vi "BioFeedback5(DAQ+FlowControl).vi"(0 "Start Trial":bool, 1 "Moving Average Length (s)":dbl=0.5, 3 "Frames Per Second":dbl=30.0, 4 "Sample rate (Hz)":dbl=1000.0, 5 "End Trial":bool, 9 "Data Directory":path, 11 "End Program":bool, 12 "File Name":string, 13 "VR Data Input File":path=path "C:/Users/Tinggroup/Desktop/VRMuscleActivationVisualizer/StationaryVisualFeedbackVR/assets/BiofeedbackData.txt", 14 "VR Percent Path":path=path "C:/Users/Tinggroup/Desktop/VRMuscleActivationVisualizer/StationaryVisualFeedbackVR/assets/BiofeedbackTargetPercentage.txt") -> (6 "Trial Data":waveform(dbl)(graph), 10 "Moving Avg RMS Graph":dbl(graph), 15 "raw data":dynamicdata(graph))   [LabVIEW 2016]
uses:
  <vilib>/Utility/error.llb/DialogType.ctl
  <vilib>/Analysis/5stat.llb/RMS (DBL).vi
  <vilib>/Waveform/WDTOps.llb/WDT Append Waveforms DBL.vi
  <vilib>/Waveform/WDTFileIO.llb/ Write Waveform to File.vi
  <vilib>/Analysis/NI_AALPro.lvlib
panel:
  in  "Extension":string="_EMG.txt"
  in  "Target Percentage":dbl
  out "Trial Data":waveform(dbl)
  out "Trial In Progress":bool
  in  "Trial Number":dbl
  in  "MARK":bool
  out "Moving Avg RMS":dbl(slide) scale=0.0..2.0
  out "Rectified Moving Average Sample":waveform(dbl)[](graph)
  out "Filtered data":waveform(dbl)
  in  "Lower Cut-Off":dbl=20.0
  in  "Upper Cut-Off":dbl=300.0
  out "Bufffer Index":dbl
  out "Frames in Buffer":dbl
  out "Samples per frame":dbl
  out "AggregateSignalData":waveform(dbl)[](array[waveform])
  out "Reset Data Acquisition\nAnd UI Updating":bool=TRUE
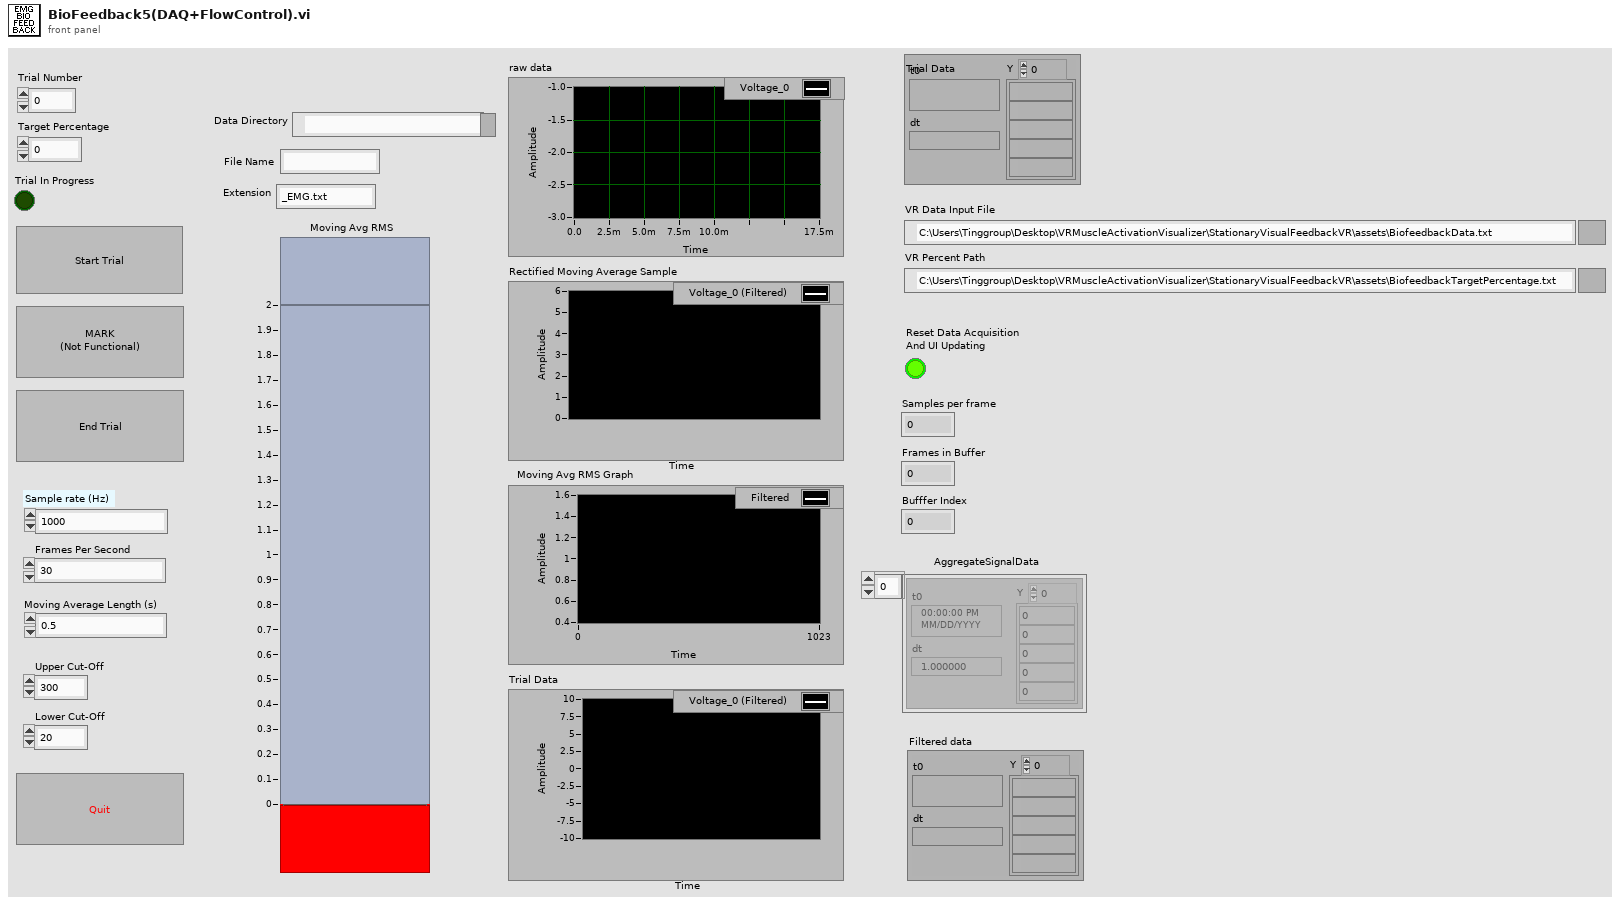
[diagram p1: front panel]
types:
  T1 = typedef "DialogType.ctl" = u16
  T2 = typedef "WaveformArrayControl.ctl" = waveform(dbl)[]
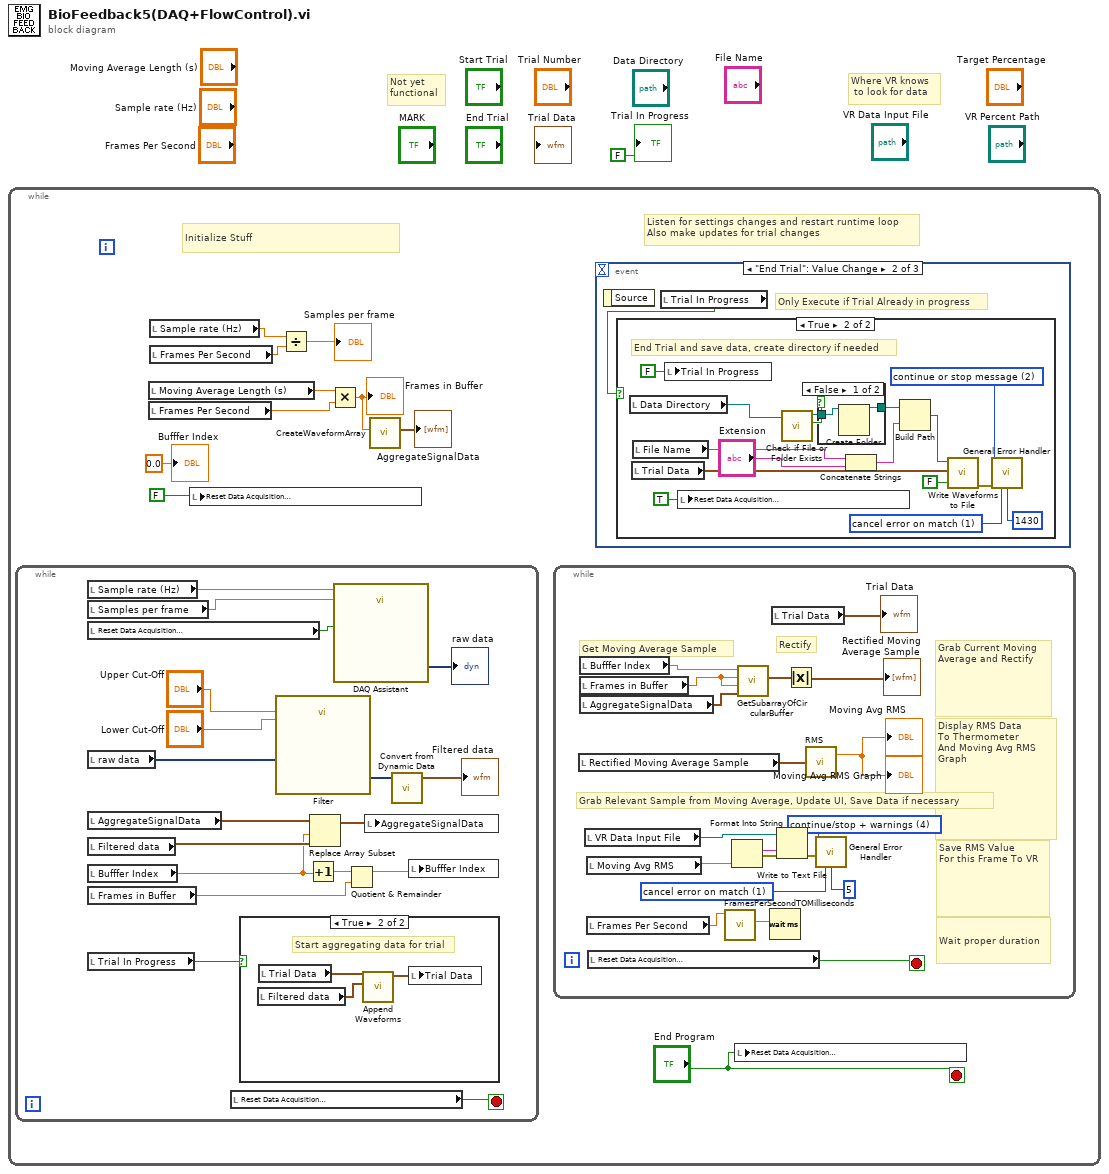
[diagram p0: block diagram]
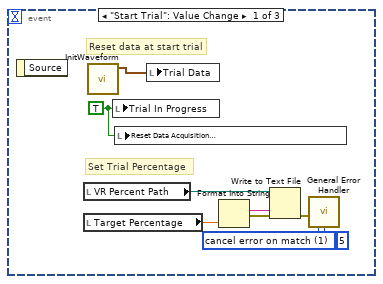
[diagram p2: hidden frame]
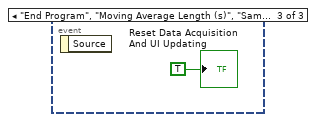
[diagram p5: hidden frame]
diagram:
  # "Not yet \nfunctional"
  # "Where VR knows\n to look for data"
  n1 = while {
    stop <- "End Program" stop-if-true
    # "Grab Relevant Sample from Moving Average, Update UI, Save Data if necessary"
    # "Initialize Stuff"
    # "Listen for settings changes and restart runtime loop\nAlso make updates for trial changes"
    n2 = while {
      stop <- w64 stop-if-true
      n3 = local read "Sample rate (Hz)"() -> (w78:dbl)
      n4 = local read "Samples per frame"() -> (w77:dbl)
      n5 = local read "Reset Data Acquisition\nAnd UI Updating"() -> (w63:bool)
      n6 = local read "raw data"() -> (w75:dynamicdata)
      n7 = local read "AggregateSignalData"() -> (w71:waveform(dbl)[])
      n8 = local read "Filtered data"() -> (w70:waveform(dbl))
      n9 = local read "Bufffer Index"() -> (w69:dbl)
      n10 = local read "Frames in Buffer"() -> (w66:dbl)
      n11 = local read "Trial In Progress"() -> (w62:bool)
      n12 = local read "Reset Data Acquisition\nAnd UI Updating"() -> (w64:bool)
      n13 = case shown="True" w62 {
        frame False {
        }
        frame True {
          # "Start aggregating data for trial"
          n14 = local read "Filtered data"() -> (w80:waveform(dbl))
          n15 = local read "Trial Data"() -> (w81:waveform(dbl))
          n16 = call-poly <vilib>:"Append Waveforms.vi"("waveform B"=w80, "waveform A"=w81) -> ("waveform out"=w79:waveform(dbl))  [unwired: 8 in, 1 out]
          n17 = local write "Trial Data"(w79) -> ()
        }
      }
      n18 = call "Filter"("Lower Cut-Off"="Lower Cut-Off", "Upper Cut-Off"="Upper Cut-Off", "Signal"=w75) -> ("Filtered Signal"=w73:dynamicdata)  [unwired: 7 in, 1 out]
      n19 = Increment(x=w69) -> (x+1=w65:dbl)
      n20 = Replace Array Subset(array=w71, new element=w70, index=w69) -> (w68:waveform(dbl)[])
      n21 = call "DAQ Assistant"("rate"=w78, "number of samples"=w77, "stop (T)"=w63) -> ("data"=→"raw data":dynamicdata)  [unwired: 14 in, 2 out]
      n22 = Quotient & Remainder(x=w65, y=w66) -> (x-y*floor(x/y)=w67:dbl)  [unwired: 1 out]
      n23 = local write "AggregateSignalData"(w68) -> ()
      n24 = call "Convert from Dynamic Data"("Dynamic Data Type"=w73) -> ("Waveform"=→"Filtered data":waveform(dbl))  [unwired: 3 in]
      n25 = local write "Bufffer Index"(w67) -> ()
    }
    n26 = local read "Moving Average Length (s)"() -> (w8:dbl)
    n27 = local read "Frames Per Second"() -> (w7:dbl)
    n28 = local read "Sample rate (Hz)"() -> (w11:dbl)
    n29 = local read "Frames Per Second"() -> (w10:dbl)
    n30 = local write "Reset Data Acquisition\nAnd UI Updating"(FALSE) -> ()
    n31 = Divide(x=w11, y=w10) -> (x/y=→"Samples per frame":dbl)
    n32 = Multiply(x=w8, y=w7) -> (x*y=w3:dbl)
    "Frames in Buffer" <- w3
    n33 = call "CreateWaveformArray.vi"("bufferSize"=w3) -> ("initialized array"=→"AggregateSignalData":waveform(dbl)[])  [unwired: 5 in, 1 out]
    n34 = while {
      stop <- w60 stop-if-true
      w42 = T1 4 items=["no dialog", "OK message", "continue or stop message", "OK message + warnings", "continue/stop + warnings"] ("type of dialog (OK msg:1)")
      w50 = 1 items=["no exception", "cancel error on match", "set error on match"] ("[exception action] (none:0)")
      # "Wait proper duration"
      # "Save RMS Value\nFor this Frame To VR"
      # "Display RMS Data\nTo Thermometer\nAnd Moving Avg RMS\nGraph"
      # "Grab Current Moving\nAverage and Rectify"
      # "Get Moving Average Sample"
      # "Rectify"
      n35 = local read "Rectified Moving Average Sample"() -> (w53:waveform(dbl)[])
      n36 = local read "Bufffer Index"() -> (w59:dbl)
      n37 = local read "Frames in Buffer"() -> (w58:dbl)
      n38 = local read "AggregateSignalData"() -> (w57:waveform(dbl)[])
      n39 = local read "VR Data Input File"() -> (w46:path)
      n40 = local read "Moving Avg RMS"() -> (w44:dbl)
      n41 = local read "Frames Per Second"() -> (w52:dbl)
      n42 = local read "Reset Data Acquisition\nAnd UI Updating"() -> (w60:bool)
      n43 = call "FramesPerSecondTOMilliseconds.vi"("Thermometer\nFps"=w52) -> ("x*y"=w51:dbl)  [unwired: 10 in]
      n44 = Format Into String(w44) -> (resulting string=w45:string, error out=w47:errorcluster)  [unwired: 3 in]
      n45 = call "GetSubarrayOfCircularBuffer.vi"("initialized array"=w57, "buffer size"=w58, "subset size"=w58, "start index"=w59) -> ("initialized array 2"=w56:T2)  [unwired: 7 in]
      n46 = Wait (ms)(milliseconds to wait=w51) -> ()  [unwired: 1 out]
      n47 = local read "Trial Data"() -> (→"Trial Data":waveform(dbl))
      n48 = Write to Text File(file (use dialog)=w46, text=w45, error in=w47) -> (error out=w48:errorcluster)  [unwired: 1 in, 2 out]
      n49 = Absolute Value(x=w56) -> (abs(x)=→"Rectified Moving Average Sample":T2)
      n50 = call-poly <vilib>:"RMS.vi"("X"=w53) -> ("rms value"=→"Moving Avg RMS" →"Moving Avg RMS Graph":dbl)  [unwired: 1 out]
      n51 = call <vilib>:"General Error Handler.vi"("type of dialog (OK msg:1)"=w42, "error in (no error)"=w48, "[exception action] (none:0)"=w50, "[exception code]"=5) -> ()  [unwired: 7 in, 5 out]
    }
    n52 = event shown="[1] \"End Trial\": Value Change" {
      selector: _ -> [_ _ _]
      dyn-events: _ -> [_ _ _]
      timeout: _ -> [_ _ _]
      event "Start Trial": Value Change {
        w18 = 1 items=["no exception", "cancel error on match", "set error on match"] ("[exception action] (none:0)")
        w19 = TRUE ("Trial In Progress")
        # "Set Trial Percentage"
        # "Reset data at start trial"
        n53 = event-data() -> ()  [unwired: 1 in, 1 out]
        n54 = local read "VR Percent Path"() -> (w13:path)
        n55 = local read "Target Percentage"() -> (w12:dbl)
        n56 = call "InitWaveform.vi"() -> ("output waveform"=w20:waveform(dbl))  [unwired: 11 in]
        n57 = local write "Trial In Progress"(w19) -> ()
        n58 = local write "Reset Data Acquisition\nAnd UI Updating"(w19) -> ()
        n59 = local write "Trial Data"(w20) -> ()
        n60 = Format Into String(w12) -> (resulting string=w14:string, error out=w15:errorcluster)  [unwired: 3 in]
        n61 = Write to Text File(file (use dialog)=w13, text=w14, error in=w15) -> (error out=w16:errorcluster)  [unwired: 1 in, 2 out]
        n62 = call <vilib>:"General Error Handler.vi"("error in (no error)"=w16, "[exception action] (none:0)"=w18, "[exception code]"=5) -> ()  [unwired: 8 in, 5 out]
      }
      event "End Trial": Value Change {
        # "Only Execute if Trial Already in progress"
        n63 = event-data() -> ()  [unwired: 1 in, 1 out]
        n64 = local read "Trial In Progress"() -> (w21:bool)
        n65 = case shown="True" w21 {
          frame False {
          }
          frame True {
            w25 = T1 2 items=["no dialog", "OK message", "continue or stop message", "OK message + warnings", "continue/stop + warnings"] ("type of dialog (OK msg:1)")
            w26 = 1 items=["no exception", "cancel error on match", "set error on match"] ("[exception action] (none:0)")
            # "End Trial and save data, create directory if needed"
            n66 = local read "Data Directory"() -> (w29:path)
            n67 = local read "Trial Data"() -> (w36:waveform(dbl))
            n68 = local read "File Name"() -> (w23:string)
            n69 = local write "Trial In Progress"(FALSE ("Trial In Progress")) -> ()
            n70 = local write "Reset Data Acquisition\nAnd UI Updating"(TRUE ("Reset Data Acquisition\nAnd UI Updating")) -> ()
            n71 = call <vilib>:"Check if File or Folder Exists.vi"("path"=w29) -> ("file or folder exists?"=w33:bool, "dup path"=w31:path)  [unwired: 8 in, 1 out]
            n72 = case shown="False" w33 {
              tunnel: [w38 w40] -> w32
              tunnel: w31 -> [w39 w40]
              frame False {
                n73 = Create Folder(path (use dialog)=w39) -> (created path=w38:path)  [unwired: 2 in, 2 out]
              }
              frame True {
              }
            }
            n74 = Concatenate Strings(w23, "Extension") -> (w22:string)
            n75 = Build Path(base path=w32, name or relative path=w22) -> (appended path=w30:path)
            n76 = call-poly <vilib>:"Write Waveforms to File.vi"("append to file? (new file:F)"=FALSE, "waveform"=w36, "file path (dialog if empty)"=w30) -> ("error out"=w28:errorcluster)  [unwired: 7 in, 1 out]
            n77 = call <vilib>:"General Error Handler.vi"("type of dialog (OK msg:1)"=w25, "error in (no error)"=w28, "[exception action] (none:0)"=w26, "[exception code]"=1430) -> ()  [unwired: 7 in, 5 out]
          }
        }
      }
      event "End Program", "Moving Average Length (s)", "Sample rate (Hz)", "Frames Per Second": Value Change {
        n78 = event-data() -> ()  [unwired: 1 in, 1 out]
        "Reset Data Acquisition\nAnd UI Updating" <- TRUE
      }
    }
    n79 = local write "Reset Data Acquisition\nAnd UI Updating"("End Program") -> ()
    "Bufffer Index" <- 0.0 ("Bufffer Index")
  }
  "Trial In Progress" <- FALSE ("Trial In Progress")
